vi "Calc Pixel Row Stats.vi"(9 "Reached Middle":bool, 10 "Reciprocals":T2, 11 "Current Row":T1) -> (1 "Row width (pixels)":sgl, 2 "Column Delta":i32, 3 "Next Row":T1, 5 "Start Col":i32, 7 "Number Of Cols This Row":i32)   [LabVIEW 2020, in "Raster (FPGA).lvlib"]
uses:
  Raster (FPGA).lvlib
  Current Row.ctl
  Reciprocals.ctl
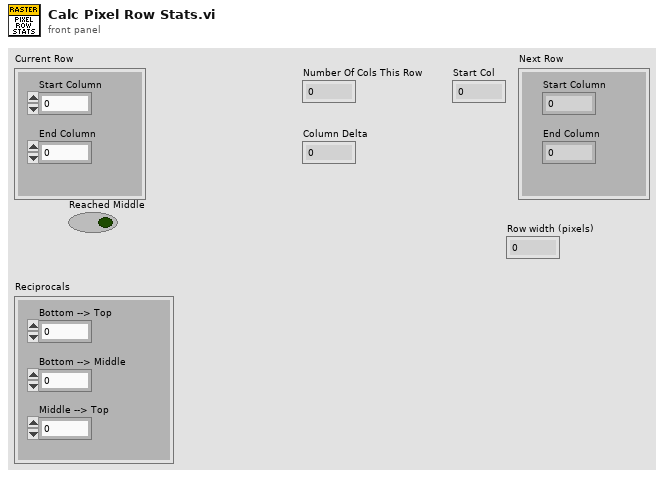
[diagram p1: front panel]
types:
  T1 = typedef "Raster (FPGA).lvlib/Current Row.ctl" = cluster{"Start Column":sgl, "End Column":sgl}
  T2 = typedef "Raster (FPGA).lvlib/Reciprocals.ctl" = cluster{"Bottom --> Top":sgl, "Bottom --> Middle":sgl, "Middle --> Top":sgl}
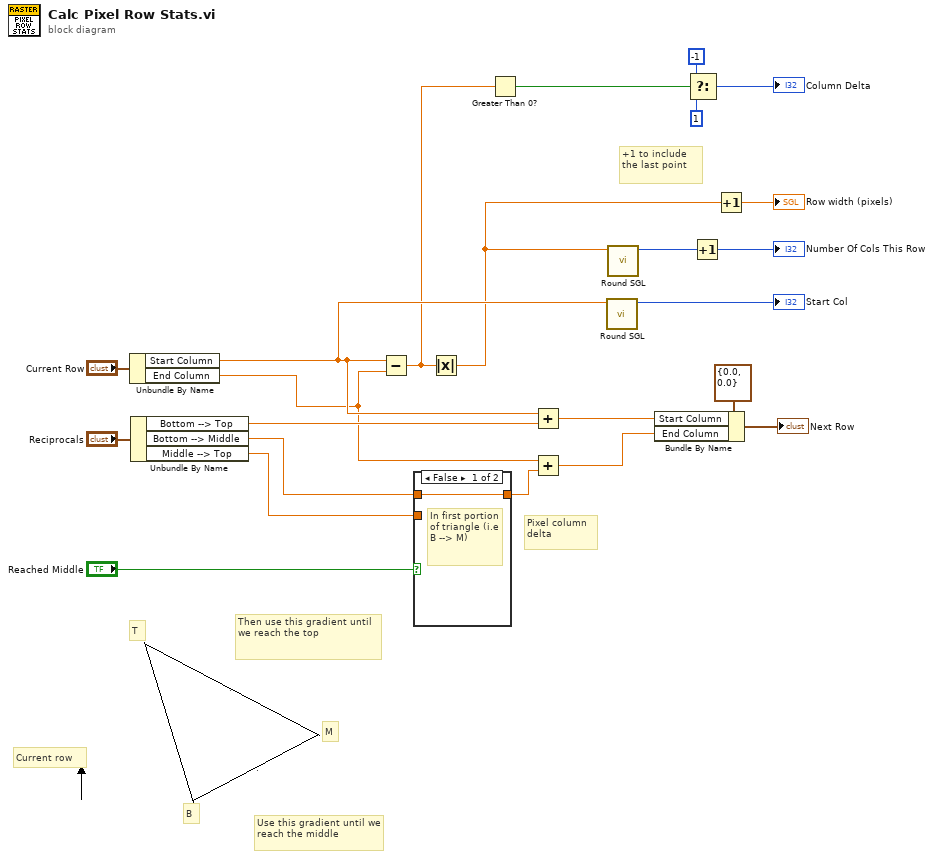
[diagram p0: block diagram]
diagram:
  # "+1 to include the last point"
  # "."
  # "."
  # "Then use this gradient until we reach the top"
  # "Use this gradient until we reach the middle"
  # "Current row"
  # "M"
  # "T"
  # "B"
  # "Pixel column delta"
  n1 = Unbundle By Name("Current Row") -> ("Start Column"=w5:sgl, "End Column"=w4:sgl)
  n2 = Unbundle By Name("Reciprocals") -> ("Bottom --> Top"=w21:sgl, "Bottom --> Middle"=w20:sgl, "Middle --> Top"=w19:sgl)
  n3 = Subtract(x=w5, y=w4) -> (x-y=w2:sgl)
  n4 = case shown="False" "Reached Middle" {
    tunnel: w20 -> [w24 _]
    tunnel: [w24 w25] -> w23
    tunnel: w19 -> [_ w25]
    frame False {
      # "In first portion of triangle (i.e B --> M)"
    }
    frame True {
      # "In second portion of triangle (i.e M --> T)"
    }
  }
  n5 = Absolute Value(x=w2) -> (abs(x)=w3:sgl)
  n6 = Greater Than 0?(x=w2) -> (x > 0?=w1:bool)
  n7 = Add(x=w5, y=w21) -> (x+y=w15:sgl)
  n8 = Add(x=w4, y=w23) -> (x+y=w14:sgl)
  n9 = call "Round SGL.vi"("SGL"=w5) -> ("I32"=→"Start Col":i32)  [unwired: 10 in]
  n10 = call "Round SGL.vi"("SGL"=w3) -> ("I32"=w7:i32)  [unwired: 10 in]
  n11 = Bundle By Name(cluster=T1 {"Start Column"=0.0, "End Column"=0.0} ("Current Row"), "Start Column"=w15, "End Column"=w14) -> (→"Next Row":T1)
  n12 = Select(t=-1 ("32bit integer"), s=w1, f=1 ("32bit integer")) -> (s? t:f=→"Column Delta":i32)
  n13 = Increment(x=w7) -> (x+1=→"Number Of Cols This Row":i32)
  n14 = Increment(x=w3) -> (x+1=→"Row width (pixels)":sgl)
